vi "Start Logic.vi"(8 "error in (no error)":errorcluster, 9 "Case name string":string, 10 "UI queue":refnum<queue>, 11 "Acq. queue in":refnum<queue>) -> (0 "error out":errorcluster, 3 "Acq. queue":refnum<queue>)   [LabVIEW 2020]
uses:
  Queue/Message Queue/Typedefs/Message Cluster.ctl
  Typedefs/PMT control functions.ctl
  Peripherals Control/Shutter/Typedefs/Shutter state.ctl
panel:
  out "Execution time (ms)":u32
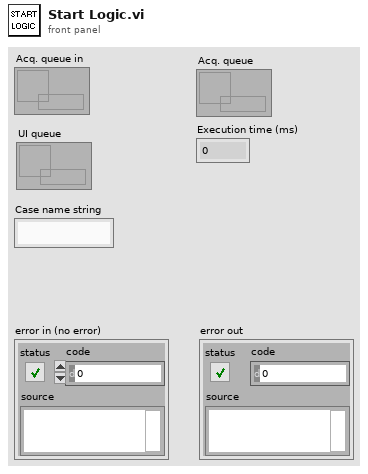
[diagram p1: front panel]
types:
  T1 = typedef "Shutter state.ctl" = enum16{"Closed/Disabled", "Open/Enabled"}
  T2 = typedef "PMT control functions.ctl" = enum16{"Set PMTs from UI", "Reset PMTs"}
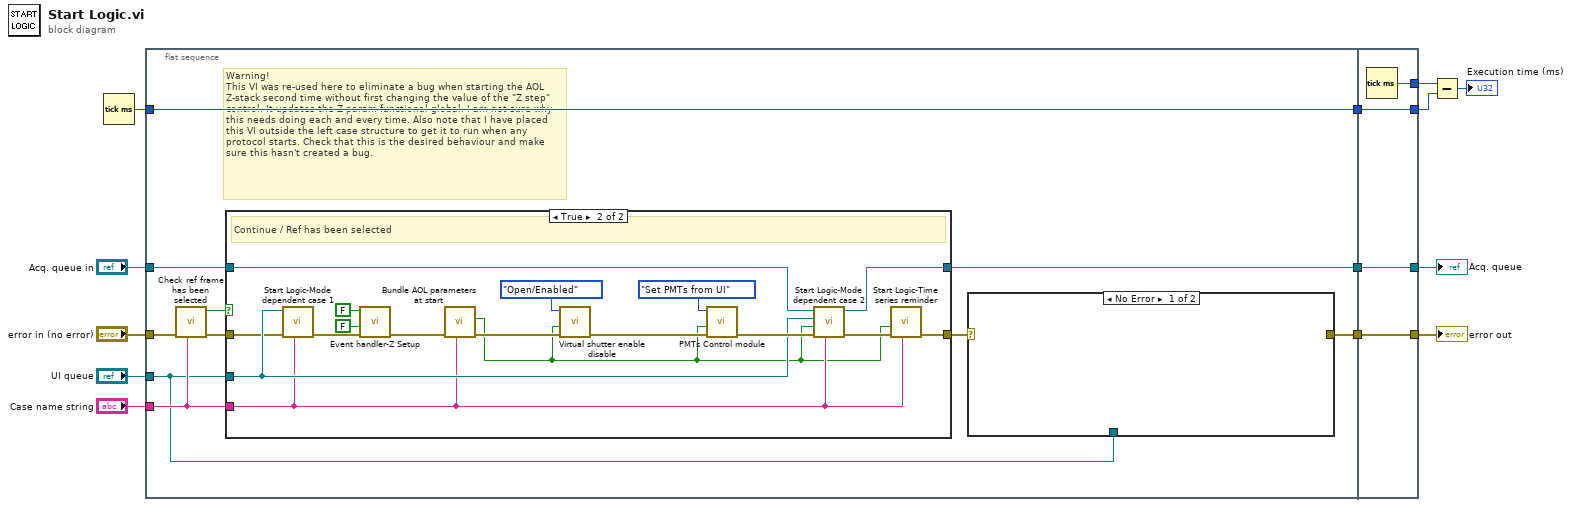
[diagram p0: block diagram]
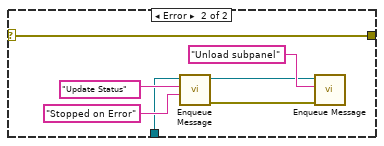
[diagram p2: hidden frame]
diagram:
  n1 = Tick Count (ms)() -> (millisecond timer value=w6:u32)
  n2 = flat-sequence {
    tunnel: "Acq. queue in" -> [w23]
    tunnel: "Case name string" -> [w19]
    tunnel: "UI queue" -> [w18]
    tunnel: "error in (no error)" -> [w15]
    tunnel: w6 -> [w14]
    tunnel: [w20] -> w5
    tunnel: [w16] -> w4
    tunnel: [w14] -> w2
    tunnel: [w52] -> w9
    tunnel: [w53] -> w12
    tunnel: w5 -> [w53]
    tunnel: w4 -> [w52]
    tunnel: [w51] -> w3
    tunnel: w2 -> [w50]
    tunnel: [w50] -> w1
    frame #0 {
      # "Warning!\nThis VI was re-used here to eliminate a bug when starting the AOL Z-stack second time without first changing the value of the \"Z step\" control. It updates the Z-param functional global. I am not sure why this needs doing each and every time. Also note that I have placed this VI outside the left case structure to get it to run when any protocol starts. Check that this is the desired behaviour and make sure this hasn't created a bug."
      n3 = call "Check ref frame has been selected.vi"("Case name string"=w19, "error in (no error)"=w15) -> ("error out"=w22:errorcluster, "Proceed / Reference frame has been selected"=w21:bool)  [unwired: 8 in]
      n4 = case shown="True" w21 {
        tunnel: [w31 w35] -> w17
        tunnel: w18 -> [_ w47]
        tunnel: w23 -> [w32 w40]
        tunnel: w19 -> [_ w34]
        tunnel: w22 -> [w31 w39]
        tunnel: [w32 w49] -> w20
        frame False {
        }
        frame True {
          # "Continue / Ref has been selected"
          n5 = call "Start Logic-Mode dependent case 1.vi"("Case name string"=w34, "error in (no error)"=w39, "UI queue"=w47) -> ("error out"=w41:errorcluster)  [unwired: 8 in]
          n6 = call "Event handler-Z Setup.vi"("error in (no error)"=w41, "Obtain Z Stop"=FALSE, "Obtain Z Start"=FALSE) -> ("error out"=w42:errorcluster)  [unwired: 8 in]
          n7 = call "Bundle AOL parameters at start.vi"("Case name string"=w34, "error in (no error)"=w42) -> ("error out"=w44:errorcluster, "cancelled"=w33:bool)  [unwired: 8 in]
          n8 = call "Virtual shutter enable disable.vi"("error in (no error)"=w44, "Cancelled"=w33, "Virtual Shutter"=Shutter_state."Open/Enabled") -> ("error out"=w43:errorcluster)  [unwired: 8 in]
          n9 = call "PMTs Control module.vi"("Error In"=w43, "Cancelled"=w33, "Function"=PMT_control_functions."Set PMTs from UI") -> ("Error Out"=w48:errorcluster)  [unwired: 8 in]
          n10 = call "Start Logic-Mode dependent case 2.vi"("Case name string"=w34, "error in (no error)"=w48, "cancelled"=w33, "UI queue"=w47, "Acq. queue in"=w40) -> ("error out"=w36:errorcluster, "Acq. queue out"=w49:refnum<queue>)  [unwired: 5 in]
          n11 = call "Start Logic-Time series reminder.vi"("Case name string"=w34, "error in (no error)"=w36, "cancelled"=w33) -> ("error out"=w35:errorcluster)  [unwired: 8 in]
        }
      }
      n12 = case shown="No Error" w17 {
        selector: w17 -> [_ w24]
        tunnel: w18 -> [_ w25]
        tunnel: [_ w24] -> w16
        frame No Error {
        }
        frame Error {
          n13 = call "Enqueue Message.vi"("Message Data"="Stopped on Error" ("Message"), "Message"="Update Status", "Queue"=w25) -> ("error out"=w27:errorcluster, "Queue out"=w26:refnum<queue>)  [unwired: 7 in]
          n14 = call "Enqueue Message.vi"("error in (no error)"=w27, "Message"="Unload subpanel", "Queue"=w26) -> ()  [unwired: 7 in, 2 out]
        }
      }
    }
    frame #1 {
      n15 = Tick Count (ms)() -> (millisecond timer value=w51:u32)
    }
  }
  n16 = Subtract(x=w3, y=w1) -> (x-y=→"Execution time (ms)":u32)
  "error out" <- w9
  "Acq. queue" <- w12
